vi "ReadRequests.vi"(8 "error in":errorcluster, 11 "condition":string) -> (0 "error out":errorcluster, 2 "Requests":T1[](array[typedef]))   [LabVIEW 2015]
uses:
  TypeDef/RequestTableCluster.ctl
  TypeDef/RequestsTableDbTableName.ctl
  <vilib>/addons/database/Connection.llb/DB Tools Open Connec (Path).vi
  <vilib>/addons/database/_DB Variant To Data/Database Variant To Data.xnode
  <vilib>/addons/database/NI_Database_API.lvlib
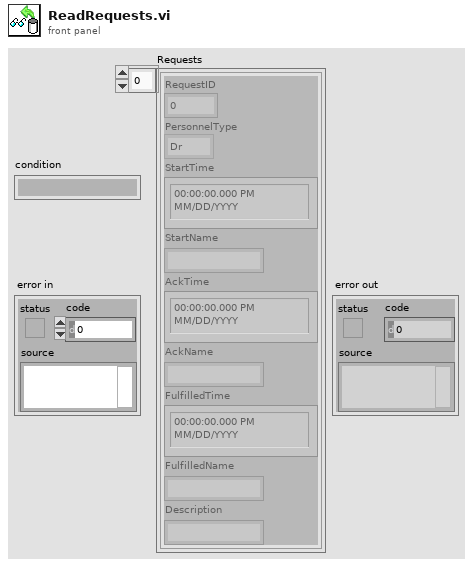
[diagram p1: front panel]
types:
  T1 = typedef "RequestTableCluster.ctl" = cluster{"RequestID":u32, "PersonnelType":enum16{"Dr", "Nurse"}, "StartTime":timestamp, "StartName":string, "AckTime":timestamp, "AckName":string, "FulfilledTime":timestamp, "FulfilledName":string, "Description":string}
  T2 = typedef "RequestsTableDbTableName.ctl" = string
  T3 = typedef "NI_Database_API.lvlib/Conn ObjectReference.ctl" = refnum<k1>
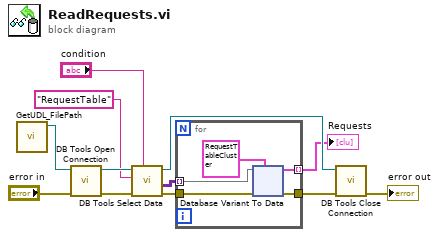
[diagram p0: block diagram]
diagram:
  n1 = call "GetUDL_FilePath.vi"() -> ("UDL file path"=w12:path)  [unwired: 11 in]
  n2 = call-poly <vilib>:"DB Tools Open Connection.vi"("error in (no error)"="error in", "connection information"=w12) -> ("error out"=w10:errorcluster, "connection reference"=w11:T3)  [unwired: 6 in]
  n3 = call <vilib>:"DB Tools Select Data.vi"("condition"="condition", "error in (no error)"=w10, "table"=T2 "RequestTable", "connection reference"=w11) -> ("error out"=w6:errorcluster, "data"=w4:variant[][], "connection reference out"=w3:T3)  [unwired: 2 in]
  n4 = for {
    tunnel: w6 -> [w17]
    tunnel: [w16] -> w5
    tunnel: w4 -> [w15] mode=indexing
    tunnel: [w13] -> w2 mode=indexing
    n5 = xnode "Database Variant To Data"("database variant"=w15, "error in (no error)"=w17, "type"=T1 {"RequestID"=0, "PersonnelType"=enum."Dr", "StartTime"=timestamp(0 s since 1904-01-01), "StartName"="", "AckTime"=timestamp(0 s since 1904-01-01), "AckName"="", "FulfilledTime"=timestamp(0 s since 1904-01-01), "FulfilledName"="", "Description"=""} ("RequestTable")) -> ("data"=w13:T1, "error out"=w16:errorcluster)
  }
  "Requests" <- w2
  n6 = call <vilib>:"DB Tools Close Connection.vi"("error in (no error)"=w5, "connection reference"=w3) -> ("error out"=→"error out":errorcluster)  [unwired: 5 in]
